vi "DataTrcFileInfo.vi"(9 "Language":u32, 11 "file path (dialog if empty)":path caption="文件路径 （空时为对话框）") -> (0 "路径输出":path, 1 "FileInfo":string, 2 "文件类型":string)   [LabVIEW 2015]
uses:
  <vilib>/Utility/file.llb/Read Delimited Spreadsheet (string).vi
  <vilib>/regexp/Match Regular Expression.xnode
panel:
  out "总帧数":i32
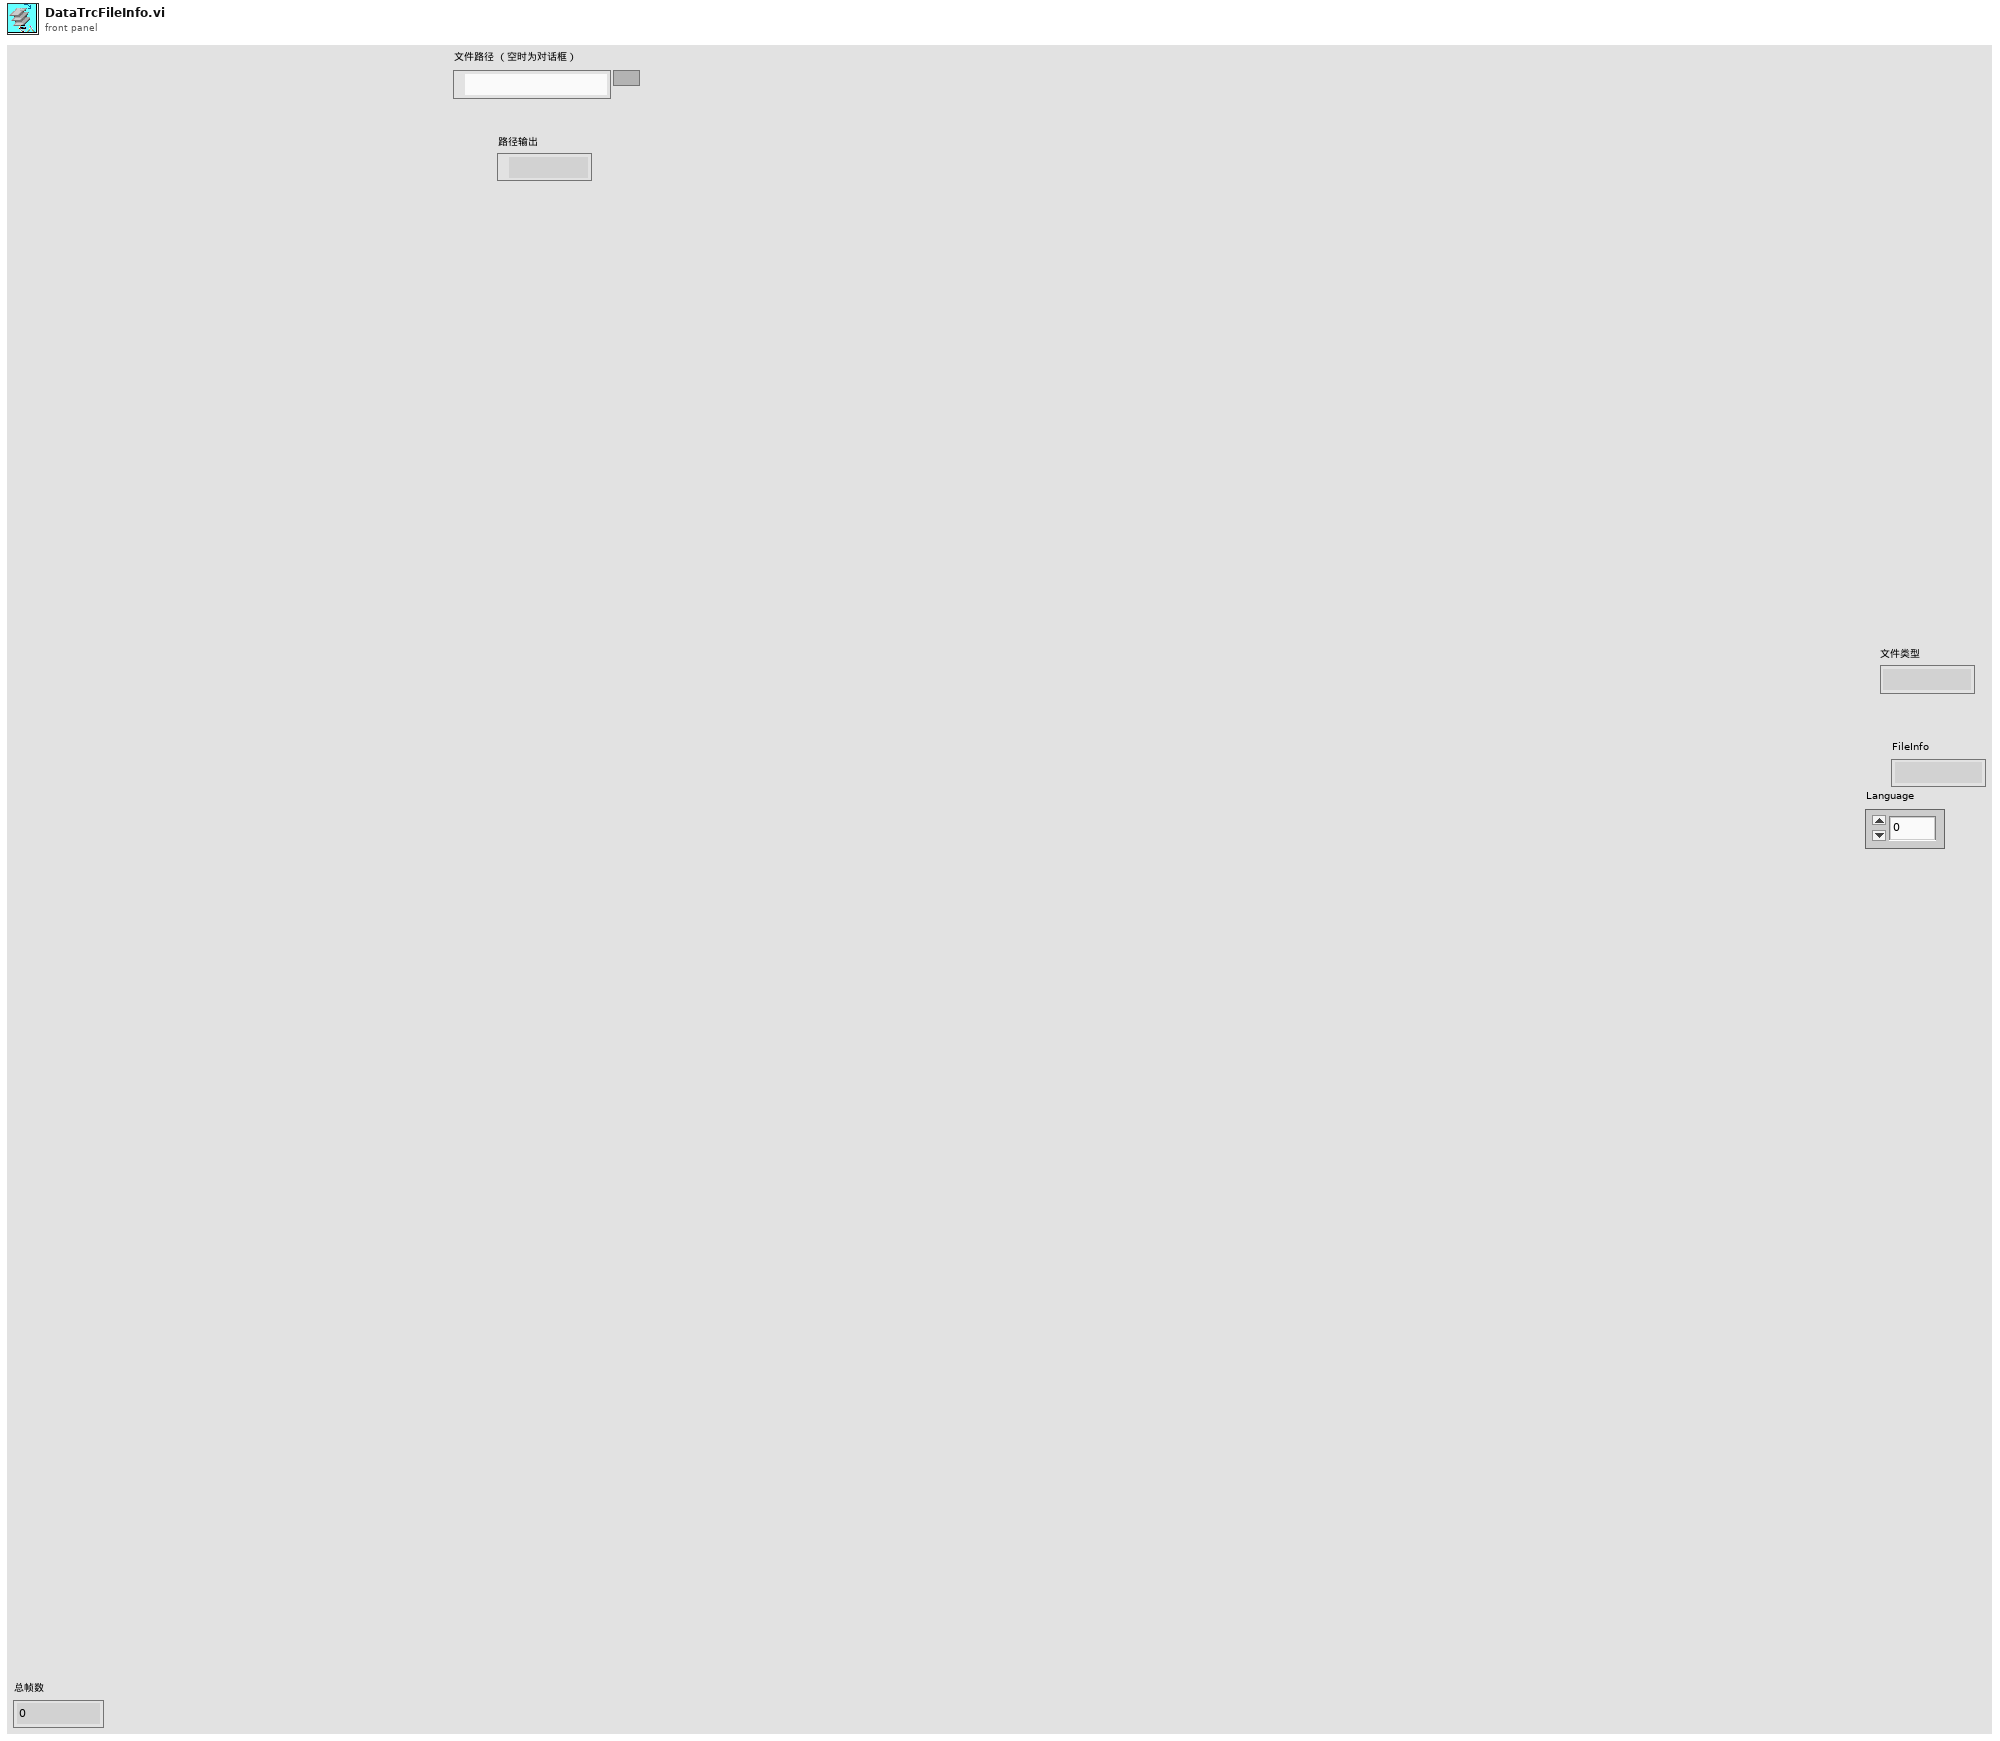
[diagram p1: front panel]
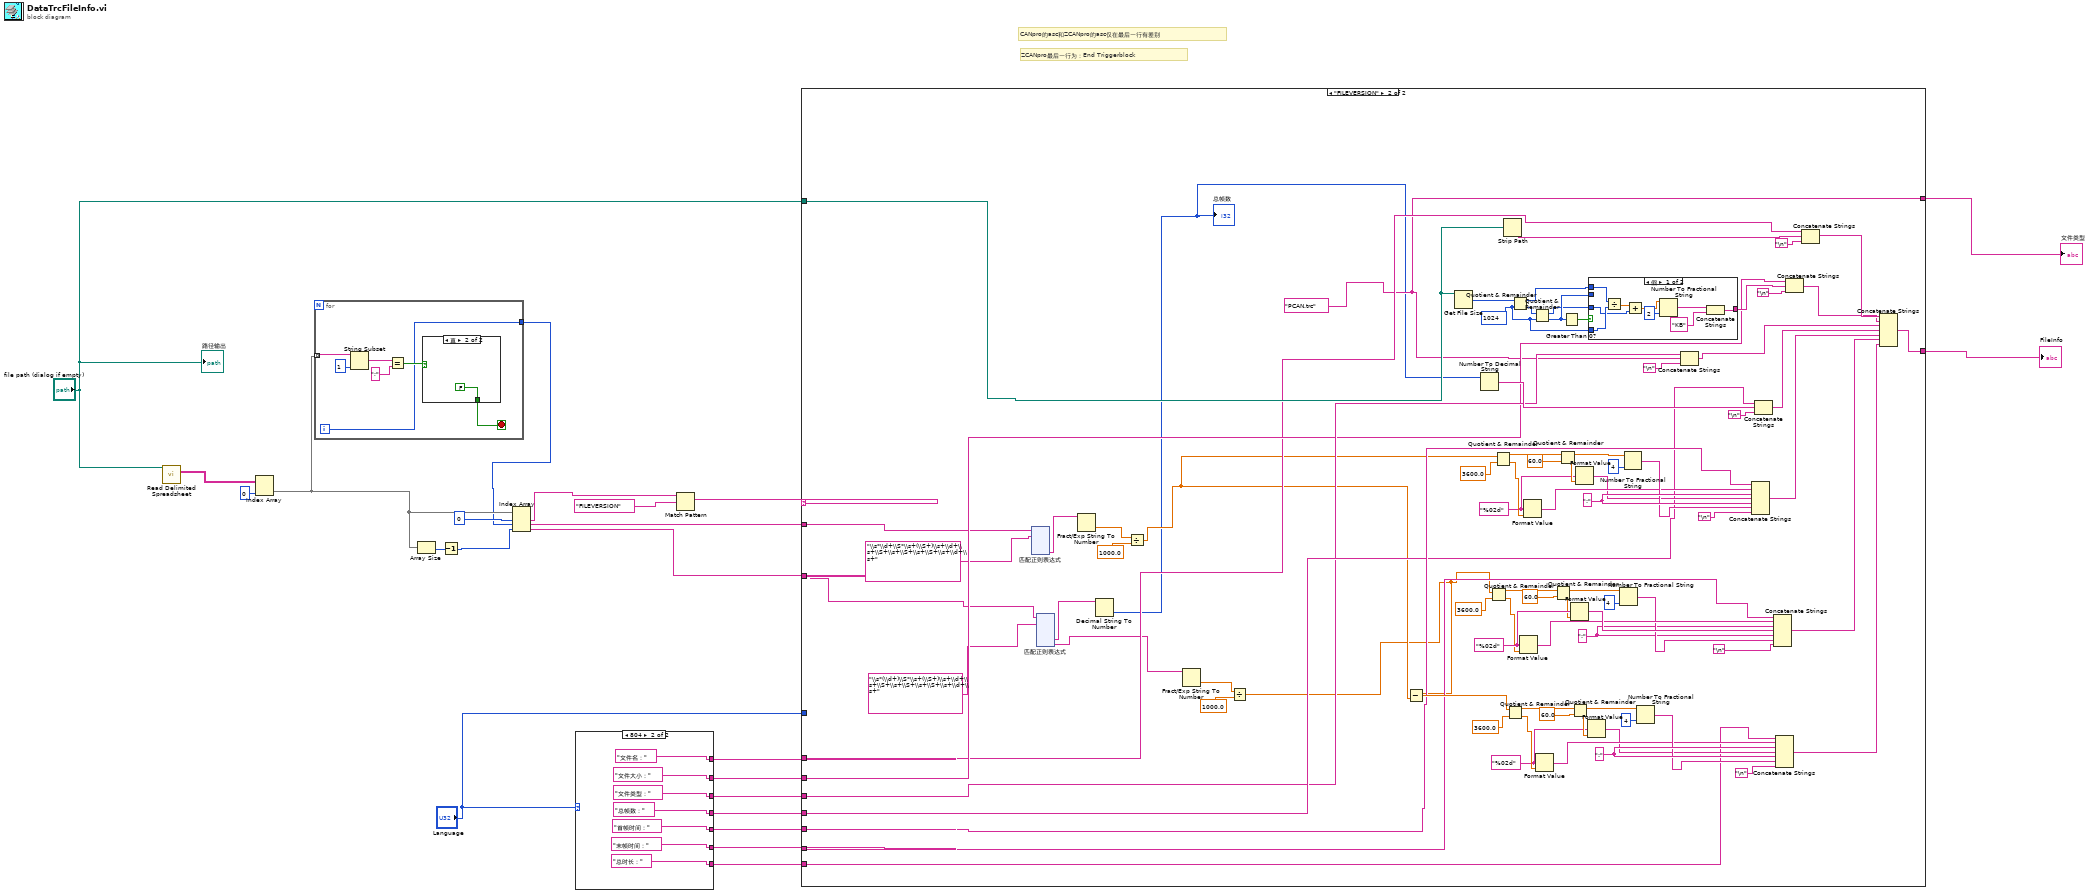
[diagram p0: block diagram]
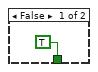
[diagram p2: hidden frame]
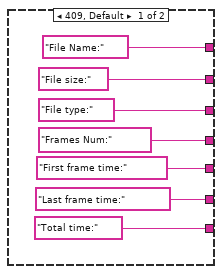
[diagram p3: hidden frame]
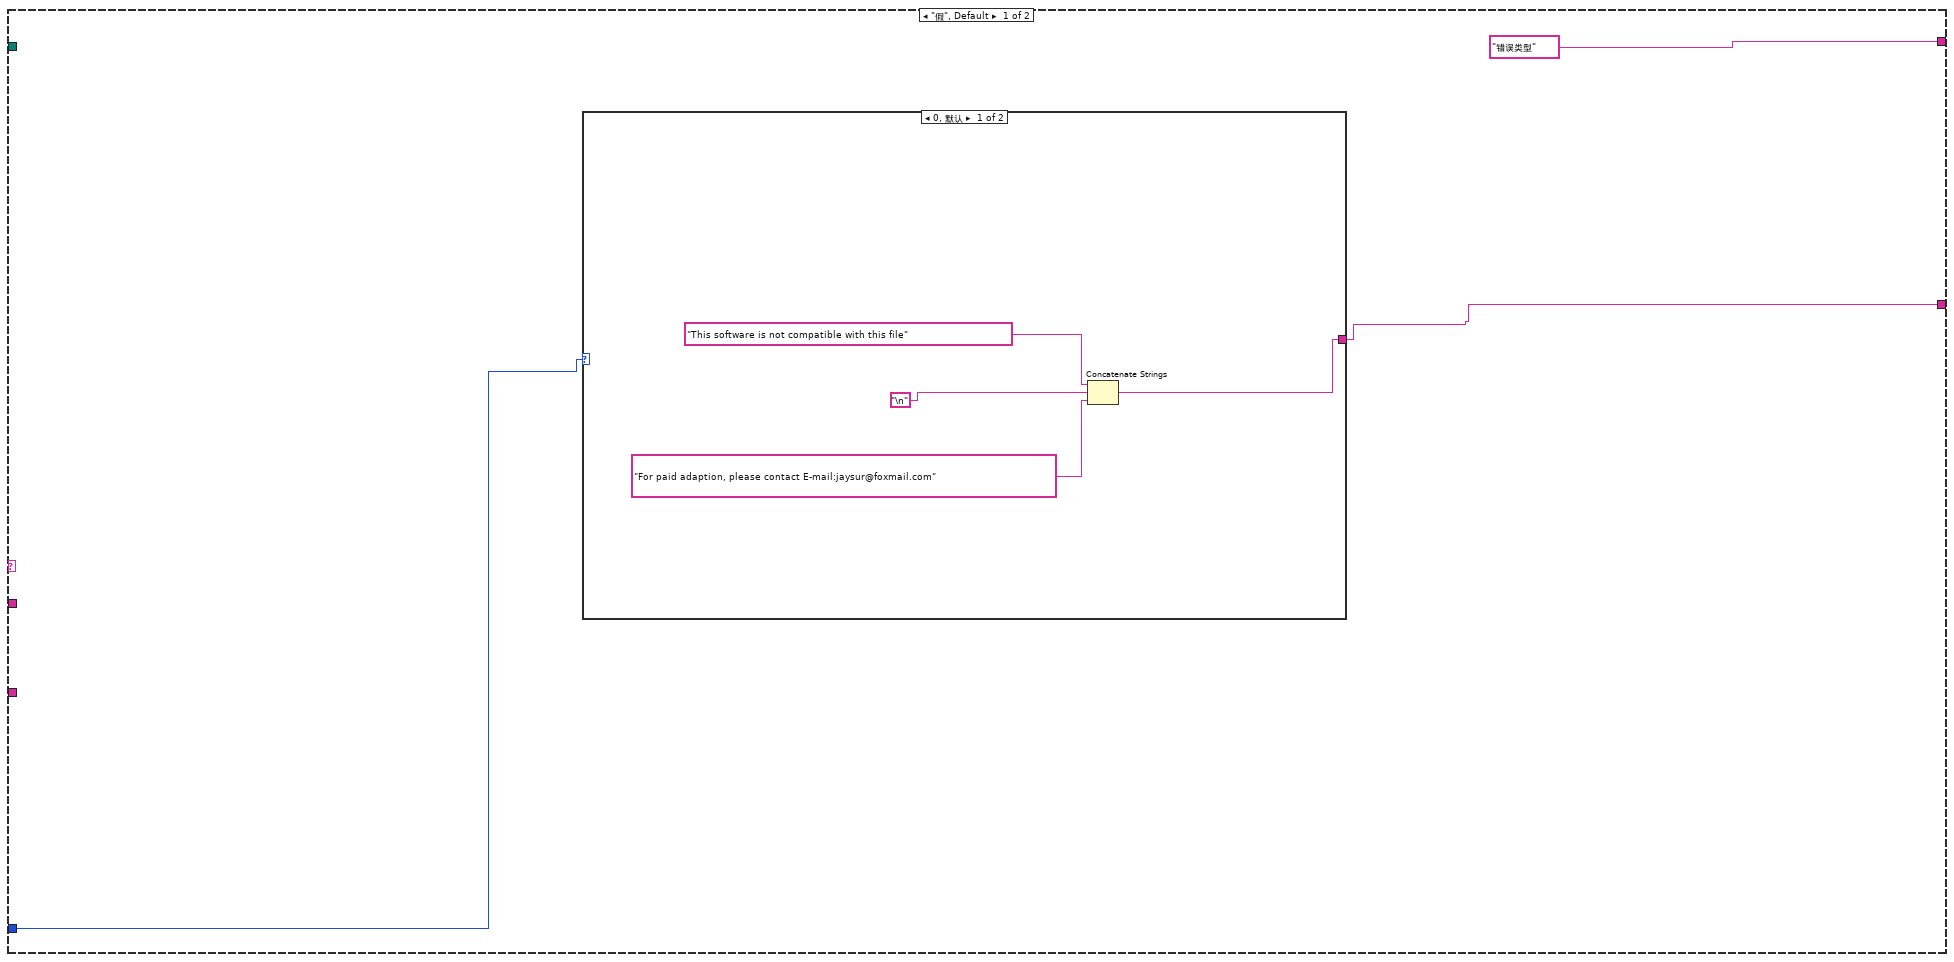
[diagram p4: hidden frame]
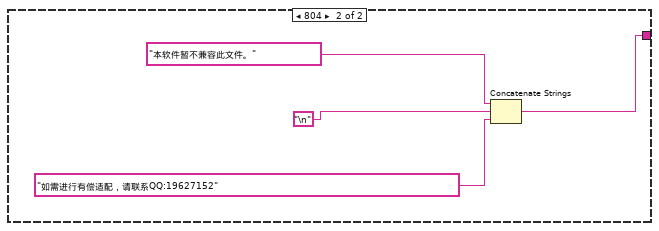
[diagram p5: hidden frame]
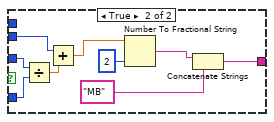
[diagram p6: hidden frame]
diagram:
  # "ZCANpro最后一行为：End Triggerblock"
  # "CANpro的asc和ZCANpro的asc仅在最后一行有差别"
  n1 = call-poly <vilib>:"Read Delimited Spreadsheet.vi"("file path (dialog if empty)"="file path (dialog if empty)") -> ("all rows"=w12:string[][])  [unwired: 9 in, 5 out]
  n2 = Index Array(array=w12, index (col)=0 ("禁用的索引 (列)")) -> (element=w2:string[])  [unwired: 1 in]
  n3 = for {
    tunnel: w2 -> [w30] mode=indexing
    tunnel: [w24] -> w1
    i -> [w24]
    stop <- w25 stop-if-true
    n4 = String Subset(string=w30, length (rest)=1 ("长度（剩余）")) -> (substring=w28:string)  [unwired: 1 in]
    n5 = Equal?(x=w28, y=";") -> (x = y?=w26:bool)
    n6 = case shown="真" w26 {
      tunnel: [TRUE FALSE] -> w25
      frame False {
      }
      frame True {
      }
    }
  }
  n7 = Array Size(array=w2) -> (size(s)=w11:i32)
  n8 = Decrement(x=w11) -> (x-1=w9:i32)
  n9 = Index Array(array=w2, index #1=0, index #2=w1, index #3=w9) -> (element #1=w7:string, element #2=w4:string, element #3=w3:string)
  n10 = case shown="804" "Language" {
    tunnel: ["Total time:" "总时长："] -> w15
    tunnel: ["Last frame time:" "末帧时间："] -> w16
    tunnel: ["First frame time:" "首帧时间："] -> w17
    tunnel: ["Frames Num:" "总帧数："] -> w18
    tunnel: ["File type:" "文件类型："] -> w19
    tunnel: ["File size:" "文件大小："] -> w20
    tunnel: ["File Name:" "文件名："] -> w21
    frame 409, Default {
    }
    frame 804 {
    }
  }
  n11 = Match Pattern(string=w7, regular expression="FILEVERSION" ("正则表达式")) -> (match substring=w5:string)  [unwired: 1 in, 3 out]
  n12 = case shown="\"FILEVERSION\"" w5 {
    tunnel: ["错误类型" w72] -> w23
    tunnel: [w48 w130] -> w22
    tunnel: "file path (dialog if empty)" -> [_ w80]
    tunnel: w21 -> [_ w73]
    tunnel: w20 -> [_ w74]
    tunnel: w19 -> [_ w75]
    tunnel: w18 -> [_ w76]
    tunnel: w17 -> [_ w77]
    tunnel: w16 -> [_ w78]
    tunnel: w15 -> [_ w79]
    tunnel: "Language" -> [w47 _]
    tunnel: w4 -> [_ w62]
    tunnel: w3 -> [_ w63]
    frame "假", Default {
      n13 = case shown="0, 默认" w47 {
        tunnel: [w50 w54] -> w48
        frame 0, Default {
          n14 = Concatenate Strings("This software is not compatible with this file", "\n", "For paid adaption, please contact E-mail:jaysur@foxmail.com") -> (w50:string)
        }
        frame 804 {
          n15 = Concatenate Strings("本软件暂不兼容此文件。", "\n", "如需进行有偿适配，请联系QQ:19627152") -> (w54:string)
        }
      }
    }
    frame "FILEVERSION" {
      w72 = "PCAN.trc"
      w85 = i64 1024 ("y")
      w104 = "%02d" ("格式字符串")
      w110 = ":"
      w128 = "%02d" ("格式字符串")
      w122 = ":"
      w131 = "%02d" ("格式字符串")
      w137 = ":"
      n16 = xnode "匹配正则表达式"("输入字符串"=w62, "正则表达式"="\\s*\\d+\\S*\\s+(\\S+)\\s+\\d+\\s+\\S+\\s+\\S+\\s+\\S+\\s+\\d+\\s+" ("格式字符串")) -> ("子匹配 1"=w70:string)  [unwired: 4 in, 5 out]
      n17 = xnode "匹配正则表达式"("输入字符串"=w63, "正则表达式"="\\s*(\\d+)\\S*\\s+(\\S+)\\s+\\d+\\s+\\S+\\s+\\S+\\s+\\S+\\s+\\d+\\s+" ("格式字符串")) -> ("子匹配 1"=w64:string, "子匹配 2"=w65:string)  [unwired: 4 in, 5 out]
      n18 = Fract/Exp String To Number(string=w70) -> (number=w69:dbl)  [unwired: 3 in, 1 out]
      n19 = Decimal String To Number(string=w64) -> (number=w59:i32)  [unwired: 2 in, 1 out]
      "总帧数" <- w59
      n20 = Divide(x=w69, y=1000.0) -> (x/y=w61:dbl)
      n21 = Fract/Exp String To Number(string=w65) -> (number=w66:dbl)  [unwired: 3 in, 1 out]
      n22 = Divide(x=w66, y=1000.0) -> (x/y=w60:dbl)
      n23 = Subtract(x=w60, y=w61) -> (x-y=w103:dbl)
      n24 = Get File Size(file=w80) -> (size (in bytes)=w88:i64)  [unwired: 1 in, 2 out]
      n25 = Number To Decimal String(number=w59) -> (decimal integer string=w91:string)  [unwired: 1 in]
      n26 = Quotient & Remainder(x=w60, y=3600.0) -> (x-y*floor(x/y)=w118:dbl, floor(x/y)=w125:dbl)
      n27 = Quotient & Remainder(x=w61, y=3600.0) -> (x-y*floor(x/y)=w141:dbl, floor(x/y)=w134:dbl)
      n28 = Strip Path(path=w80) -> (name=w98:string)  [unwired: 1 out]
      n29 = Quotient & Remainder(x=w103, y=3600.0) -> (x-y*floor(x/y)=w114:dbl, floor(x/y)=w107:dbl)
      n30 = Quotient & Remainder(x=w88, y=w85) -> (x-y*floor(x/y)=w81:i64, floor(x/y)=w87:i64)
      n31 = Format Value(format string=w128, value (0)=w125) -> (output string=w124:string)  [unwired: 1 in]
      n32 = Format Value(format string=w131, value (0)=w134) -> (output string=w135:string)  [unwired: 1 in]
      n33 = Quotient & Remainder(x=w87, y=w85) -> (x-y*floor(x/y)=w83:i64, floor(x/y)=w84:i64)
      n34 = Format Value(format string=w104, value (0)=w107) -> (output string=w108:string)  [unwired: 1 in]
      n35 = Quotient & Remainder(x=w118, y=60.0) -> (x-y*floor(x/y)=w120:dbl, floor(x/y)=w126:dbl)
      n36 = Quotient & Remainder(x=w141, y=60.0) -> (x-y*floor(x/y)=w139:dbl, floor(x/y)=w133:dbl)
      n37 = Greater Than 0?(x=w84) -> (x > 0?=w86:bool)
      n38 = Format Value(format string=w128, value (0)=w126) -> (output string=w127:string)  [unwired: 1 in]
      n39 = Quotient & Remainder(x=w114, y=60.0) -> (x-y*floor(x/y)=w112:dbl, floor(x/y)=w106:dbl)
      n40 = Format Value(format string=w131, value (0)=w133) -> (output string=w132:string)  [unwired: 1 in]
      n41 = Format Value(format string=w104, value (0)=w106) -> (output string=w105:string)  [unwired: 1 in]
      n42 = case shown="假" w86 {
        tunnel: w85 -> [w381 w391]
        tunnel: w84 -> [_ w389]
        tunnel: w83 -> [w379 w392]
        tunnel: [w384 w387] -> w82
        tunnel: w81 -> [w382 _]
        frame False {
          n43 = Divide(x=w382, y=w381) -> (x/y=w380:dbl)
          n44 = Add(x=w380, y=w379) -> (x+y=w378:dbl)
          n45 = Number To Fractional String(number=w378, precision (6)=i16 2 ("精度(6)")) -> (F-format string=w376:string)  [unwired: 2 in]
          n46 = Concatenate Strings(w376, "KB" ("字符串")) -> (w384:string)
        }
        frame True {
          n47 = Divide(x=w392, y=w391) -> (x/y=w390:dbl)
          n48 = Add(x=w389, y=w390) -> (x+y=w388:dbl)
          n49 = Number To Fractional String(number=w388, precision (6)=i16 2 ("精度(6)")) -> (F-format string=w386:string)  [unwired: 2 in]
          n50 = Concatenate Strings(w386, "MB") -> (w387:string)
        }
      }
      n51 = Number To Fractional String(number=w120, precision (6)=i16 4 ("精度(6)")) -> (F-format string=w123:string)  [unwired: 2 in]
      n52 = Number To Fractional String(number=w139, precision (6)=i16 4 ("精度(6)")) -> (F-format string=w136:string)  [unwired: 2 in]
      n53 = Number To Fractional String(number=w112, precision (6)=i16 4 ("精度(6)")) -> (F-format string=w109:string)  [unwired: 2 in]
      n54 = Concatenate Strings(w75, w72, "\n") -> (w95:string)
      n55 = Concatenate Strings(w77, w135, w137, w132, w137, w136, "\n") -> (w129:string)
      n56 = Concatenate Strings(w76, w91, "\n") -> (w92:string)
      n57 = Concatenate Strings(w78, w124, w122, w127, w122, w123, "\n") -> (w116:string)
      n58 = Concatenate Strings(w79, w108, w110, w105, w110, w109, "\n") -> (w102:string)
      n59 = Concatenate Strings(w74, w82, "\n") -> (w89:string)
      n60 = Concatenate Strings(w73, w98, "\n") -> (w97:string)
      n61 = Concatenate Strings(w97, w89, w95, w92, w129, w116, w102) -> (w130:string)
    }
  }
  "FileInfo" <- w22
  "文件类型" <- w23
  "路径输出" <- "file path (dialog if empty)"
